vi "Get Tab Ctrl Number.vi"(11 "CtlRef":refnum<vi>) -> (2 "number":u32)   [LabVIEW 2011]
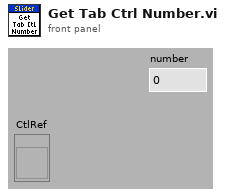
[diagram p1: front panel]
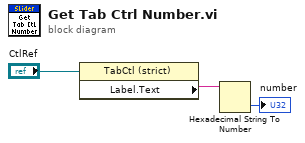
[diagram p0: block diagram]
diagram:
  n1 = property class="TabCtl (strict)"(reference="CtlRef") -> ("Label.Text"=w2:string)  [unwired: 1 in, 2 out]
  n2 = Hexadecimal String To Number(string=w2) -> (number=→"number":u32)  [unwired: 3 out]
